vi "Sub.vi"   [LabVIEW 2014]
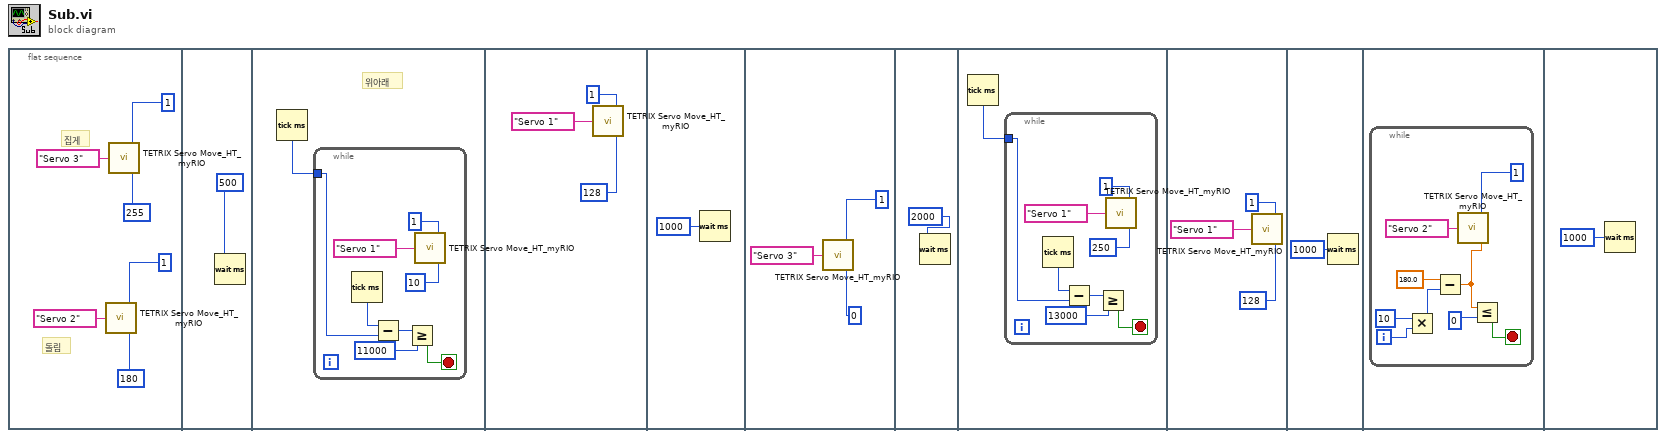
[diagram p0: block diagram]
diagram:
  n1 = flat-sequence {
    frame #0 {
      # "돌림"
      # "집게"
      n2 = call <vilib>:"TETRIX Servo Move_HT_myRIO.vi"("Servo Position (0 - 255)"=u8 180, "Controller Daisy Chain Position (1 - 4)"=u8 1, "Select Servo"="Servo 2") -> ()  [unwired: 2 in, 1 out]
      n3 = call <vilib>:"TETRIX Servo Move_HT_myRIO.vi"("Servo Position (0 - 255)"=u8 255, "Controller Daisy Chain Position (1 - 4)"=u8 1, "Select Servo"="Servo 3") -> ()  [unwired: 2 in, 1 out]
    }
    frame #1 {
      n4 = Wait (ms)(milliseconds to wait=u32 500 ("대기 시간(ms)")) -> ()  [unwired: 1 out]
    }
    frame #2 {
      # "위아래"
      n5 = Tick Count (ms)() -> (millisecond timer value=w8:u32)
      n6 = while {
        tunnel: w8 -> [w12]
        stop <- w10 stop-if-true
        n7 = Tick Count (ms)() -> (millisecond timer value=w13:u32)
        n8 = Subtract(x=w13, y=w12) -> (x-y=w11:u32)
        n9 = Greater Or Equal?(x=w11, y=u32 11000) -> (x >= y?=w10:bool)
        n10 = call <vilib>:"TETRIX Servo Move_HT_myRIO.vi"("Servo Position (0 - 255)"=u8 10, "Controller Daisy Chain Position (1 - 4)"=u8 1, "Select Servo"="Servo 1") -> ()  [unwired: 2 in, 1 out]
      }
    }
    frame #3 {
      n11 = call <vilib>:"TETRIX Servo Move_HT_myRIO.vi"("Servo Position (0 - 255)"=u8 128, "Controller Daisy Chain Position (1 - 4)"=u8 1, "Select Servo"="Servo 1") -> ()  [unwired: 2 in, 1 out]
    }
    frame #4 {
      n12 = Wait (ms)(milliseconds to wait=u32 1000 ("대기 시간(ms)")) -> ()  [unwired: 1 out]
    }
    frame #5 {
      n13 = call <vilib>:"TETRIX Servo Move_HT_myRIO.vi"("Servo Position (0 - 255)"=u8 0, "Controller Daisy Chain Position (1 - 4)"=u8 1, "Select Servo"="Servo 3") -> ()  [unwired: 2 in, 1 out]
    }
    frame #6 {
      n14 = Wait (ms)(milliseconds to wait=u32 2000 ("ms 타이머 값")) -> ()  [unwired: 1 out]
    }
    frame #7 {
      n15 = Tick Count (ms)() -> (millisecond timer value=w25:u32)
      n16 = while {
        tunnel: w25 -> [w29]
        stop <- w27 stop-if-true
        n17 = Tick Count (ms)() -> (millisecond timer value=w30:u32)
        n18 = Subtract(x=w30, y=w29) -> (x-y=w28:u32)
        n19 = Greater Or Equal?(x=w28, y=u32 13000) -> (x >= y?=w27:bool)
        n20 = call <vilib>:"TETRIX Servo Move_HT_myRIO.vi"("Servo Position (0 - 255)"=u8 250, "Controller Daisy Chain Position (1 - 4)"=u8 1, "Select Servo"="Servo 1") -> ()  [unwired: 2 in, 1 out]
      }
    }
    frame #8 {
      n21 = call <vilib>:"TETRIX Servo Move_HT_myRIO.vi"("Servo Position (0 - 255)"=u8 128, "Controller Daisy Chain Position (1 - 4)"=u8 1, "Select Servo"="Servo 1") -> ()  [unwired: 2 in, 1 out]
    }
    frame #9 {
      n22 = Wait (ms)(milliseconds to wait=u32 1000 ("대기 시간(ms)")) -> ()  [unwired: 1 out]
    }
    frame #10 {
      n23 = while {
        i -> [w42]
        stop <- w39 stop-if-true
        n24 = Multiply(x=10, y=w42) -> (x*y=w43:i32)
        n25 = Subtract(x=180.0, y=w43) -> (x-y=w38:dbl)
        n26 = call <vilib>:"TETRIX Servo Move_HT_myRIO.vi"("Servo Position (0 - 255)"=w38, "Controller Daisy Chain Position (1 - 4)"=u8 1, "Select Servo"="Servo 2") -> ()  [unwired: 2 in, 1 out]
        n27 = Less Or Equal?(x=w38, y=u8 0 ("Servo Position (0 - 255)")) -> (x <= y?=w39:bool)
      }
    }
    frame #11 {
      n28 = Wait (ms)(milliseconds to wait=u32 1000 ("대기 시간(ms)")) -> ()  [unwired: 1 out]
    }
  }
